vi "sendCommand.vi"(6 "Axis Letter":string, 8 "error in (no error)":errorcluster, 9 "Value":string, 10 "Command":string, 11 "Controller in":refnum<class "Controller.lvclass">) -> (0 "error out":errorcluster, 3 "Controller out":refnum<class "Controller.lvclass">)   [LabVIEW 2019, in "Controller.lvclass"]
uses:
  Controller.lvclass
  Controller.lvclass/Controller.ctl
  Communication/Communication.lvclass
  Axis/Axis.lvclass
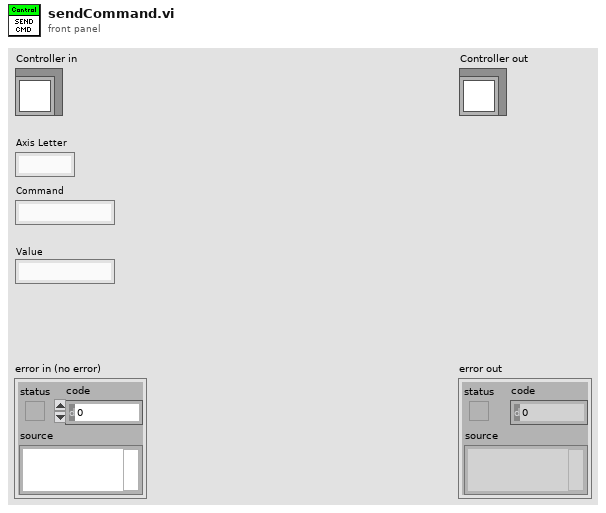
[diagram p1: front panel]
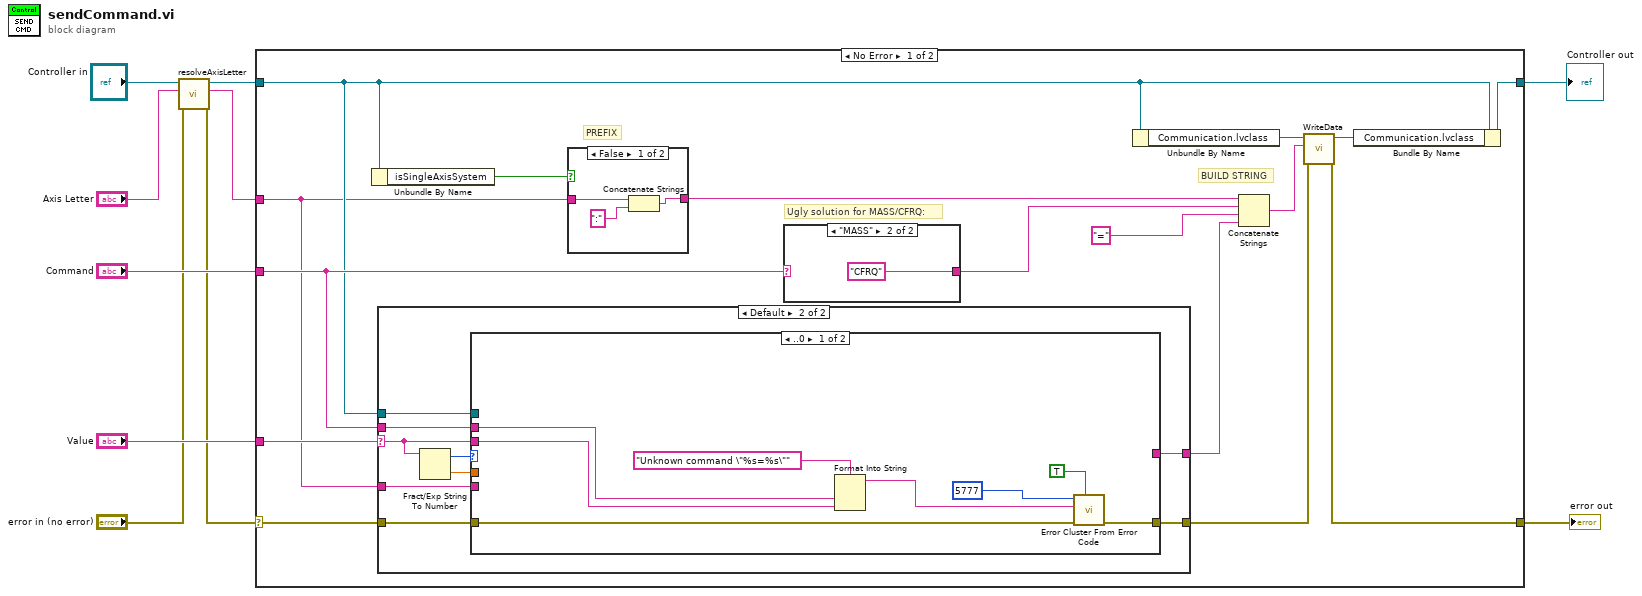
[diagram p0: block diagram]
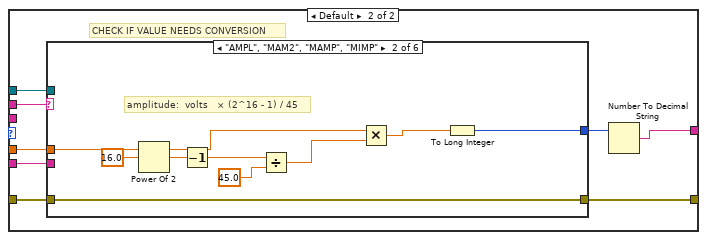
[diagram p3: hidden frame]
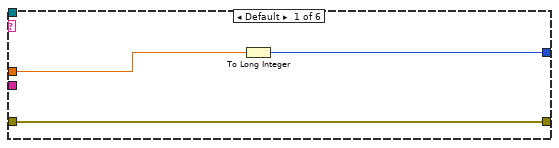
[diagram p4: hidden frame]
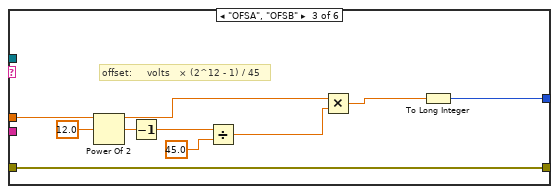
[diagram p5: hidden frame]
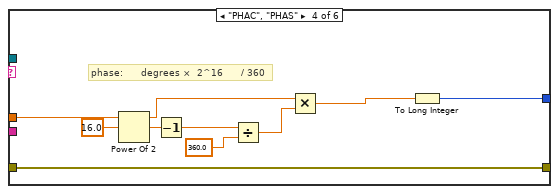
[diagram p6: hidden frame]
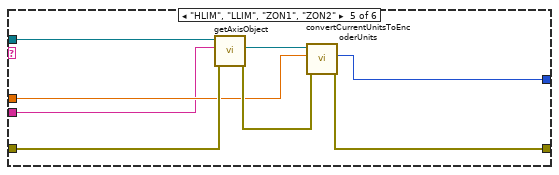
[diagram p7: hidden frame]
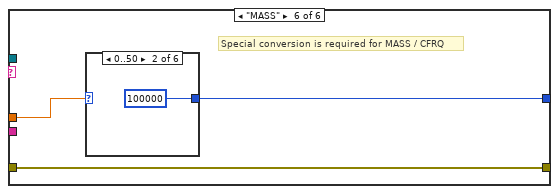
[diagram p8: hidden frame]
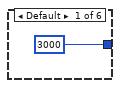
[diagram p9: hidden frame]
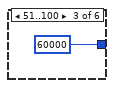
[diagram p10: hidden frame]
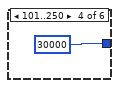
[diagram p11: hidden frame]
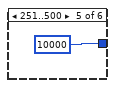
[diagram p12: hidden frame]
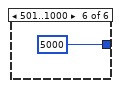
[diagram p13: hidden frame]
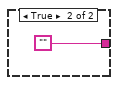
[diagram p14: hidden frame]
diagram:
  n1 = call "resolveAxisLetter.vi"("error in (no error)"="error in (no error)", "Axis Letter in"="Axis Letter", "Controller in"="Controller in") -> ("error out"=w3:errorcluster, "Axis Letter out"=w1:string, "Controller out"=w5:refnum<class "Controller.lvclass">)  [unwired: 6 in]
  n2 = case shown="No Error" w3 {
    selector: w3 -> [w14 w108]
    tunnel: [w18 w108] -> w10
    tunnel: [w19 w107] -> w9
    tunnel: w5 -> [w13 w107]
    tunnel: "Command" -> [w15 _]
    tunnel: w1 -> [w12 _]
    tunnel: "Value" -> [w16 _]
    frame No Error {
      # "Ugly solution for MASS/CFRQ:"
      # "BUILD STRING"
      # "PREFIX"
      n3 = Unbundle By Name(w13) -> ("isSingleAxisSystem"=w26:bool)
      n4 = case shown="Default" w16 {
        selector: w16 -> [w28 w29]
        tunnel: [w28 w37] -> w20
        tunnel: w12 -> [_ w36]
        tunnel: w15 -> [_ w35]
        tunnel: w14 -> [w27 w34]
        tunnel: w13 -> [_ w33]
        tunnel: [w27 w30] -> w11
        frame "?" {
        }
        frame Default {
          n5 = Fract/Exp String To Number(string=w29) -> (offset past number=w31:i32, number=w32:dbl)  [unwired: 3 in]
          n6 = case shown="..0" w31 {
            tunnel: [_ w53] -> w37
            tunnel: w36 -> [_ w52]
            tunnel: w35 -> [w41 w51]
            tunnel: w34 -> [w44 w49]
            tunnel: w33 -> [_ w48]
            tunnel: w32 -> [_ w47]
            tunnel: [w45 w46] -> w30
            tunnel: w29 -> [w40 _]
            frame ..0 {
              n7 = Format Into String(format string="Unknown command \"%s=%s\"" ("error message (\"\")"), w41, w40) -> (resulting string=w38:string)  [unwired: 2 in, 1 out]
              n8 = call <vilib>:"Error Cluster From Error Code.vi"("show call chain? (False)"=TRUE, "error in (no error)"=w44, "error message (\"\")"=w38, "error code (0)"=5777) -> ("error out"=w45:errorcluster)  [unwired: 5 in]
            }
            frame Default {
              # "CHECK IF VALUE NEEDS CONVERSION"
              n9 = case shown="\"AMPL\", \"MAM2\", \"MAMP\", \"MIMP\"" w51 {
                tunnel: w47 -> [w56 w65 w74 w83 w87 w94]
                tunnel: [w55 w58 w72 w76 w86 w93] -> w50
                tunnel: w48 -> [_ _ _ _ w90 _]
                tunnel: w49 -> [w54 w57 w66 w75 w89 w92]
                tunnel: w52 -> [_ _ _ _ w85 _]
                tunnel: [w54 w57 w66 w75 w84 w92] -> w46
                frame Default {
                  n10 = To Long Integer(number=w56) -> (32bit integer=w55:i32)
                }
                frame "AMPL", "MAM2", "MAMP", "MIMP" {
                  # "amplitude:  volts   × (2^16 - 1) / 45"
                  n11 = Power Of 2(x=16.0) -> (2^x=w61:dbl)
                  n12 = Decrement(x=w61) -> (x-1=w60:dbl)
                  n13 = Divide(x=w60, y=45.0) -> (x/y=w59:dbl)
                  n14 = Multiply(x=w65, y=w59) -> (x*y=w64:dbl)
                  n15 = To Long Integer(number=w64) -> (32bit integer=w58:i32)
                }
                frame "OFSA", "OFSB" {
                  # "offset:     volts   × (2^12 - 1) / 45"
                  n16 = Power Of 2(x=12.0) -> (2^x=w68:dbl)
                  n17 = Decrement(x=w68) -> (x-1=w67:dbl)
                  n18 = Divide(x=w67, y=45.0) -> (x/y=w70:dbl)
                  n19 = Multiply(x=w74, y=w70) -> (x*y=w73:dbl)
                  n20 = To Long Integer(number=w73) -> (32bit integer=w72:i32)
                }
                frame "PHAC", "PHAS" {
                  # "phase:      degrees ×  2^16      / 360"
                  n21 = Power Of 2(x=16.0) -> (2^x=w79:dbl)
                  n22 = Decrement(x=w79) -> (x-1=w78:dbl)
                  n23 = Divide(x=w78, y=360.0) -> (x/y=w77:dbl)
                  n24 = Multiply(x=w83, y=w77) -> (x*y=w82:dbl)
                  n25 = To Long Integer(number=w82) -> (32bit integer=w76:i32)
                }
                frame "HLIM", "LLIM", "ZON1", "ZON2" {
                  n26 = call-dynamic "getAxisObject.vi"("error in (no error)"=w89, "Axis Letter"=w85, "Controller in"=w90) -> ("error out"=w91:errorcluster, "Axis Object"=w88:refnum<class "Axis.lvclass">)  [unwired: 6 in, 1 out]
                  n27 = call-dynamic "convertCurrentUnitsToEncoderUnits.vi"("error in (no error)"=w91, "Value In Current Units"=w87, "Axis in"=w88) -> ("error out"=w84:errorcluster, "Value In Encoder Units"=w86:i32)  [unwired: 6 in, 1 out]
                }
                frame "MASS" {
                  # "Special conversion is required for MASS / CFRQ"
                  n28 = case shown="0..50" w94 {
                    tunnel: [3000 100000 60000 30000 10000 5000] -> w93
                    frame Default {
                    }
                    frame 0..50 {
                    }
                    frame 51..100 {
                    }
                    frame 101..250 {
                    }
                    frame 251..500 {
                    }
                    frame 501..1000 {
                    }
                  }
                }
              }
              n29 = Number To Decimal String(number=w50) -> (decimal integer string=w53:string)  [unwired: 1 in]
            }
          }
        }
      }
      n30 = case shown="False" w26 {
        tunnel: w12 -> [w103 _]
        tunnel: [w102 ""] -> w25
        frame False {
          n31 = Concatenate Strings(w103, ":") -> (w102:string)
        }
        frame True {
        }
      }
      n32 = case shown="\"MASS\"" w15 {
        selector: w15 -> [w105 _]
        tunnel: [w105 "CFRQ"] -> w21
        frame Default {
        }
        frame "MASS" {
        }
      }
      n33 = Unbundle By Name(w13) -> ("Communication.lvclass"=w23:refnum<class "Communication.lvclass">)
      n34 = Concatenate Strings(w25, w21, "=", w20) -> (w17:string)
      n35 = call-dynamic "WriteData.vi"("error in (no error)"=w11, "DataToWrite"=w17, "Communication in"=w23) -> ("error out"=w18:errorcluster, "Communication out"=w22:refnum<class "Communication.lvclass">)  [unwired: 7 in]
      n36 = Bundle By Name(cluster=w13, "Communication.lvclass"=w22) -> (w19:refnum<class "Controller.lvclass">)
    }
    frame Error {
    }
  }
  "error out" <- w10
  "Controller out" <- w9
